vi "Event Handle Loop_Mini Panel.vi"(8 "error in (no error)":errorcluster, 11 "QTab Class in":refnum<class "QTab Class.lvclass">) -> (0 "error out":errorcluster, 2 "OK?":bool, 3 "QTab Class Out":refnum<class "QTab Class.lvclass">)   [LabVIEW 2020, in "QTab.lvlib" / "QTab Class.lvclass"]
uses:
  QTab Class.lvclass
  <vilib>/Utility/miscctls.llb/LVRectTypeDef.ctl
  QTab Class.lvclass/QTab Class.ctl
panel:
  out "Picture":picture
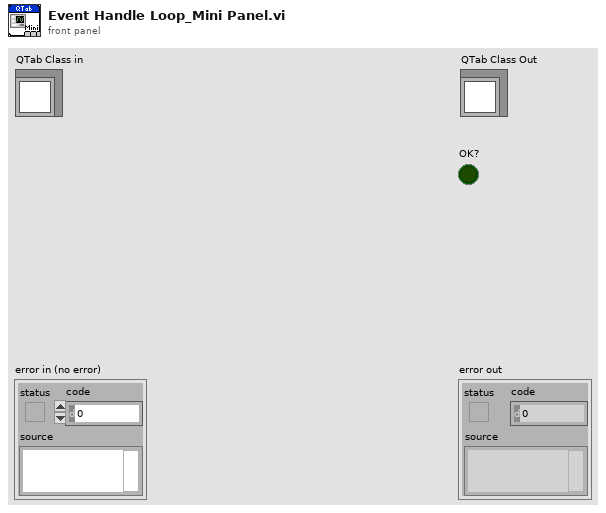
[diagram p1: front panel]
types:
  T1 = enum32{"Invalid", "Standard", "Closed", "Hidden", "Minimized", "Maximized"}
  T2 = typedef "LVRectTypeDef.ctl" = cluster{"Left":i16, "Top":i16, "Right":i16, "Bottom":i16}
  T3 = typedef "imagedata.ctl" = cluster{"image type":i32, "image depth":i32, "image":u8[], "mask":u8[], "colors":u32[], "Rectangle":cluster{"left":i16, "top":i16, "right":i16, "bottom":i16}}
  T4 = typedef "LVPoint32TypeDef.ctl" = cluster{"Horizontal":i32, "Vertical":i32}
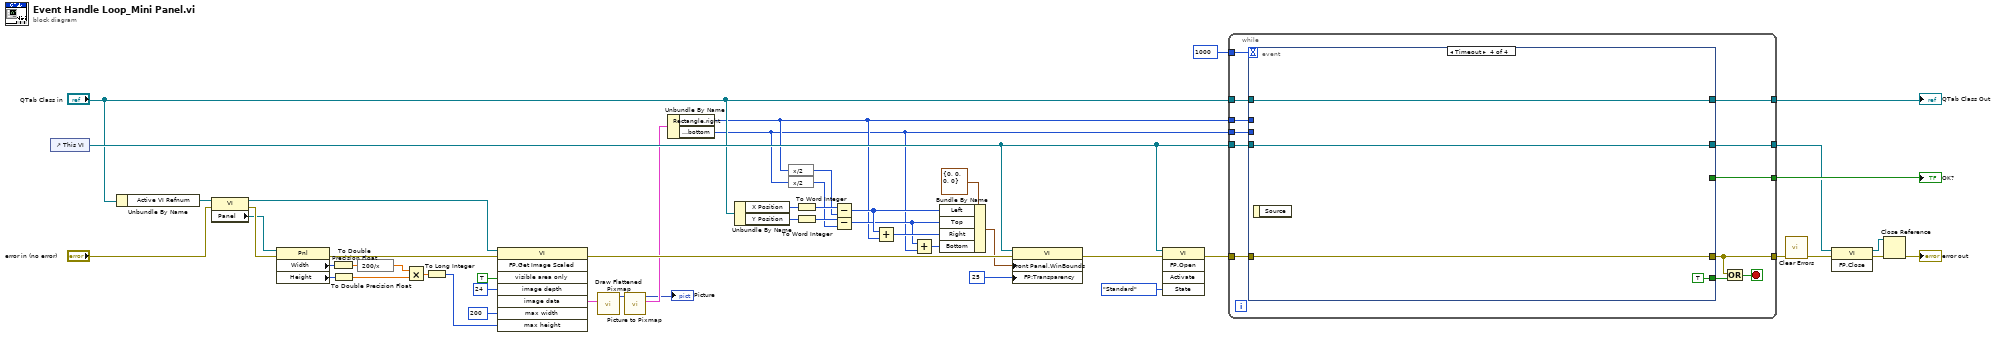
[diagram p0: block diagram]
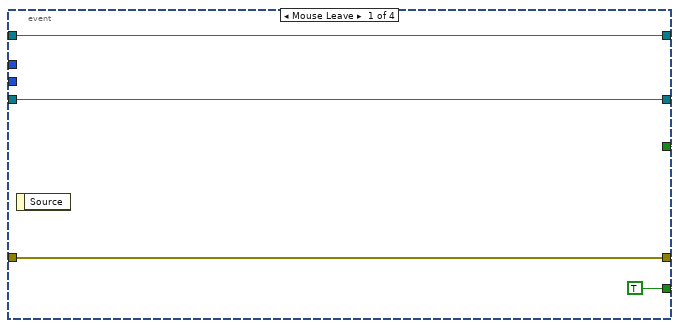
[diagram p2: hidden frame]
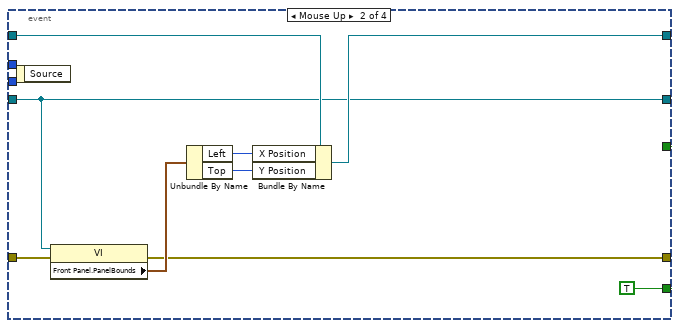
[diagram p3: hidden frame]
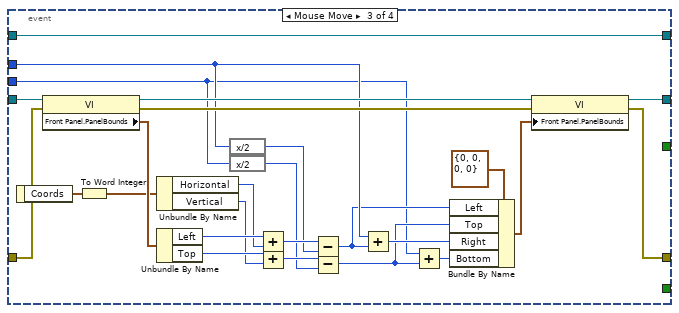
[diagram p4: hidden frame]
diagram:
  n1 = control-ref of="This VI"() -> (w48:refnum<vi>)
  n2 = Unbundle By Name("QTab Class in") -> ("Active VI Refnum"=w32:refnum<vi>)
  n3 = property class="VI"(reference=w32, error in="error in (no error)") -> (reference out=w24:refnum<vi>, error out=w35:errorcluster, "Panel"=w34:refnum<vi>)
  n4 = property class="Pnl"(reference=w34, error in=w35) -> (error out=w33:errorcluster, "Width"=w30:u32, "Height"=w29:u32)  [unwired: 1 out]
  n5 = To Double Precision Float(number=w30) -> (double precision float=w31:dbl)
  n6 = To Double Precision Float(number=w29) -> (double precision float=w28:dbl)
  n7 = expression code="200/x"(w31) -> (w27:dbl)
  n8 = Multiply(x=w27, y=w28) -> (x*y=w26:dbl)
  n9 = To Long Integer(number=w26) -> (32bit integer=w25:i32)
  n10 = invoke class="VI" method="FP.Get Image Scaled"(reference=w24, error in=w33, "visible area only"=TRUE ("Visible Area Only"), "image depth"=24 ("Image Depth"), "max width"=200 ("Maximum Width"), "max height"=w25) -> (error out=w42:errorcluster, "image data"=w44:T3)  [unwired: 2 in, 6 out]
  n11 = call <vilib>:"Draw Flattened Pixmap.vi"("image data"=w44) -> ("new picture"=w43:picture)  [unwired: 8 in]
  n12 = call <vilib>:"Picture to Pixmap.vi"("picture"=w43) -> ("image data"=w41:T3, "new picture"=→"Picture":picture)  [unwired: 9 in]
  n13 = Unbundle By Name(w41) -> ("Rectangle.right"=w8:i16, "Rectangle.bottom"=w7:i16)
  n14 = Unbundle By Name("QTab Class in") -> ("X Position"=w23:i16, "Y Position"=w22:i16)
  n15 = expression code="x/2"(w8) -> (w14:i16)
  n16 = expression code="x/2"(w7) -> (w12:i16)
  n17 = To Word Integer(number=w23) -> (16bit integer=w15:i16)
  n18 = To Word Integer(number=w22) -> (16bit integer=w13:i16)
  n19 = Subtract(x=w15, y=w14) -> (x-y=w11:i16)
  n20 = Subtract(x=w13, y=w12) -> (x-y=w9:i16)
  n21 = Add(x=w11, y=w8) -> (x+y=w10:i16)
  n22 = Add(x=w9, y=w7) -> (x+y=w39:i16)
  n23 = Bundle By Name(cluster=T2 {"Left"=0, "Top"=0, "Right"=0, "Bottom"=0} ("Front Panel Window:Window Bounds"), "Left"=w11, "Top"=w9, "Right"=w10, "Bottom"=w39) -> (w36:T2)
  n24 = property class="VI"(reference=w48, error in=w42, "Front Panel.WinBounds"=w36, "FP:Transparency"=u8 25 ("Front Panel Window:Transparency")) -> (error out=w21:errorcluster)  [unwired: 1 out]
  n25 = invoke class="VI" method="FP.Open"(reference=w48, error in=w21, "State"=T1."Standard") -> (error out=w20:errorcluster)  [unwired: 2 in, 4 out]
  n26 = while {
    tunnel: [w54] -> w2
    tunnel: w20 -> [w62]
    tunnel: w48 -> [w61]
    tunnel: "QTab Class in" -> [w60]
    tunnel: w8 -> [w59]
    tunnel: w7 -> [w58]
    tunnel: [w57] -> w50
    tunnel: [w56] -> w49
    tunnel: [w52] -> w3
    tunnel: 1000 -> [w51]
    stop <- w53 stop-if-true
    n27 = event shown="[3] Timeout" {
      selector: _ -> [_ _ _ _]
      dyn-events: _ -> [_ _ _ _]
      timeout: w51 -> [_ _ _ _]
      tunnel: w62 -> [w63 w74 w100 w103]
      tunnel: [w63 w67 w91 w103] -> w54
      tunnel: w61 -> [w64 w70 w101 w104]
      tunnel: w60 -> [w65 w72 w86 w105]
      tunnel: [w66 w75 _ TRUE] -> w55
      tunnel: w59 -> [_ _ w83 _]
      tunnel: w58 -> [_ _ w76 _]
      tunnel: [w65 w71 w86 w105] -> w57
      tunnel: [w66 w75 _ _] -> w56
      tunnel: [w64 w70 w85 w104] -> w52
      event Mouse Leave {
        w66 = TRUE
        n28 = event-data() -> ()  [unwired: 1 in, 1 out]
      }
      event Mouse Up {
        w75 = TRUE
        n29 = event-data() -> ()  [unwired: 1 in, 1 out]
        n30 = property class="VI"(reference=w70, error in=w74) -> (error out=w67:errorcluster, "Front Panel.PanelBounds"=w73:T2)  [unwired: 1 out]
        n31 = Unbundle By Name(w73) -> ("Left"=w69:i16, "Top"=w68:i16)
        n32 = Bundle By Name(cluster=w72, "X Position"=w69, "Y Position"=w68) -> (w71:refnum<class "QTab Class.lvclass">)
      }
      event Mouse Move {
        n33 = event-data() -> ("Coords"=w98:T4)  [unwired: 1 in]
        n34 = property class="VI"(reference=w101, error in=w100) -> (reference out=w93:refnum<vi>, error out=w92:errorcluster, "Front Panel.PanelBounds"=w99:T2)
        n35 = To Word Integer(number=w98) -> (16bit integer=w97:cluster{"Horizontal":i16, "Vertical":i16})
        n36 = Unbundle By Name(w97) -> ("Horizontal"=w84:i16, "Vertical"=w94:i16)
        n37 = Unbundle By Name(w99) -> ("Left"=w96:i16, "Top"=w95:i16)
        n38 = expression code="x/2"(w83) -> (w81:i16)
        n39 = expression code="x/2"(w76) -> (w79:i16)
        n40 = Add(x=w96, y=w84) -> (x+y=w82:i16)
        n41 = Add(x=w95, y=w94) -> (x+y=w80:i16)
        n42 = Subtract(x=w82, y=w81) -> (x-y=w78:i16)
        n43 = Subtract(x=w80, y=w79) -> (x-y=w77:i16)
        n44 = Add(x=w83, y=w78) -> (x+y=w89:i16)
        n45 = Add(x=w76, y=w77) -> (x+y=w88:i16)
        n46 = Bundle By Name(cluster=T2 {"Left"=0, "Top"=0, "Right"=0, "Bottom"=0} ("Front Panel Window:Window Bounds"), "Left"=w78, "Top"=w77, "Right"=w89, "Bottom"=w88) -> (w87:T2)
        n47 = property class="VI"(reference=w93, error in=w92, "Front Panel.PanelBounds"=w87) -> (reference out=w85:refnum<vi>, error out=w91:errorcluster)
      }
      event Timeout {
        n48 = event-data() -> ()  [unwired: 1 in, 1 out]
      }
    }
    n49 = Or(x=w54, y=w55) -> (x .or. y?=w53:bool)
  }
  "QTab Class Out" <- w50
  "OK?" <- w49
  n50 = call <vilib>:"Clear Errors.vi"("error in (no error)"=w2) -> ("error out"=w1:errorcluster)  [unwired: 5 in, 1 out]
  n51 = invoke class="VI" method="FP.Close"(reference=w3, error in=w1) -> (reference out=w4:refnum<vi>, error out=w5:errorcluster)  [unwired: 1 in, 1 out]
  n52 = Close Reference(reference=w4, error in (no error)=w5) -> (error out=→"error out":errorcluster)
